vi "数值与布尔转换.vi"() -> ()   [LabVIEW 2023]
doc: "本VI是为《我和LabVIEW》一书编写的示例。\n关于本书的介绍请参考网页：\nhttp://ruanqizhen.spaces.live.com/blog/cns!5852D4F797C53FB6!4310.entry"
panel:
  out "I16数值":i16
  out "布尔":bool
  out "数值":i32
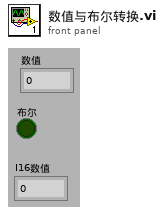
[diagram p1: front panel]
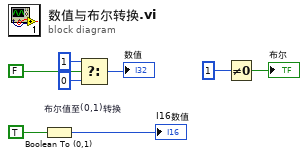
[diagram p0: block diagram]
diagram:
  n1 = Boolean To (0,1) "布尔值至(0,1)转换"(Boolean=TRUE) -> (0, 1=→"I16数值":i16)
  n2 = Select(t=1, s=FALSE, f=0) -> (s? t:f=→"数值":i32)
  n3 = Not Equal To 0?(x=1) -> (x != 0?=→"布尔":bool)
